vi "Force Variable.vi"(0 "variable path (URL)":string, 5 "forced value":variant, 11 "error in (no error)":errorcluster) -> (15 "error out":errorcluster)   [LabVIEW 2017]
doc: "Forces an I/O variable or I/O alias to assume <B>forced value</B> until you disable forcing, reboot the target, or force the variable to assume a new <B>forced value</B>."
uses:
  <resource>/objmgr/ni.var.rc
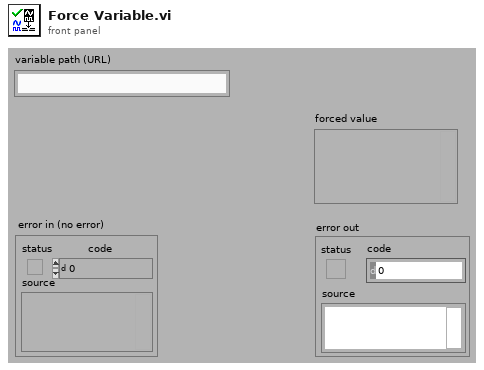
[diagram p1: front panel]
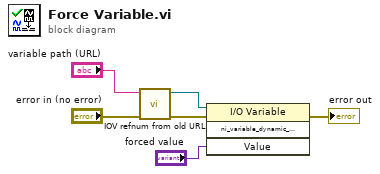
[diagram p0: block diagram]
diagram:
  n1 = call <vilib>:"IOV refnum from old URL.vi"("error in (no error)"="error in (no error)", "variable path (URL)"="variable path (URL)") -> ("error out"=w2:errorcluster, "IOV refnum"=w1:refnum<k21>)  [unwired: 8 in]
  n2 = invoke class="I/O Variable" method="ni_variable_dynamic_IOVariable_Force"(reference=w1, error in=w2, "Value"="forced value") -> (error out=→"error out":errorcluster)  [unwired: 1 in, 3 out]
